vi "Destroy.vi"   [LabVIEW 2018, in "Toolkit.lvlib" / "Agent.lvclass"]
doc: "Destroys an existing Agent object. This deallocates, or frees, the resources in the libssh2 library that were allocated when the Agent object was created. An Agent object must not be used after it is destroyed; otherwise, LabVIEW could crash."
uses:
  Agent.lvclass
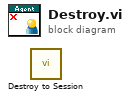
[diagram p0: block diagram]
diagram:
  n1 = call "Destroy to Session.vi"() -> ()  [unwired: 10 in, 2 out]
